vi "TW Convert Top Level.vi"() -> ()   [LabVIEW 2021, in "Plugin Generator.lvlib"]
uses:
  Plugin Generator.lvlib
panel:
  out "error out":errorcluster
  in  "Text color":u32(colorbox)
  in  "Background":u32(colorbox)=14457856
  in  "New Name":string="CIFRocks"
  in  "Template Project Path":path=path "D:/dev/Plugins/CIF_ROCKS/Tests/Template Interactive Test.lvproj"
  in  "Icon Text":string="RK-ON"
  # "To do:\nUpdate UI proj (will break after update)\nUpdate OOB test project\nUpdate Build Library project"
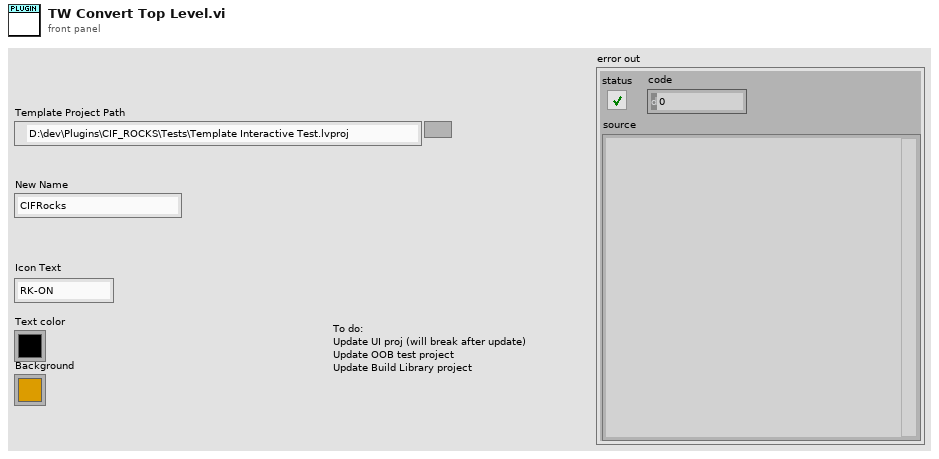
[diagram p1: front panel]
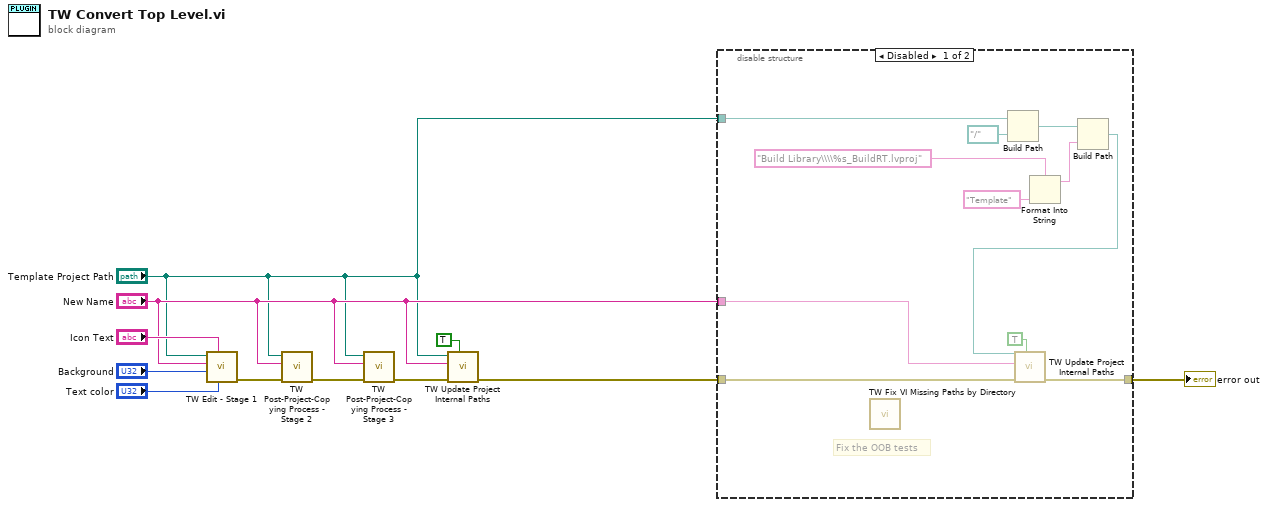
[diagram p0: block diagram]
diagram:
  n1 = call "TW Edit - Stage 1.vi"("Text color"="Text color", "Icon Text"="Icon Text", "Background"="Background", "New Subname"="New Name", "Template Project Path"="Template Project Path") -> ("error out"=w8:errorcluster)  [unwired: 5 in, 1 out]
  n2 = call "TW Post-Project-Copying Process - Stage 2.vi"("error in"=w8, "New Subname"="New Name", "Template Project Path"="Template Project Path") -> ("error out"=w7:errorcluster)  [unwired: 8 in]
  n3 = call "TW Post-Project-Copying Process - Stage 3.vi"("error in"=w7, "New Subname"="New Name", "Template Project Path"="Template Project Path") -> ("error out"=w6:errorcluster)  [unwired: 8 in]
  n4 = call "TW Update Project Internal Paths.vi"("Rename Project"=TRUE, "error in (no error)"=w6, "New Subname"="New Name", "Project Path"="Template Project Path") -> ("error out"=w4:errorcluster)  [unwired: 7 in]
  n5 = disable-structure shown="Disabled" {
    disable-tunnel: w4 -> [w22 w23]
    disable-tunnel: "New Name" -> [w21 _]
    disable-tunnel: [w12 w23] -> w2
    disable-tunnel: "Template Project Path" -> [w14 _]
    frame Disabled {
      # "Fix the OOB tests"
      n6 = call "TW Fix VI Missing Paths by Directory.vi"() -> ()  [unwired: 11 in, 1 out]
      n7 = Build Path(base path=w14, name or relative path=path "../..") -> (appended path=w16:path)
      n8 = Format Into String(format string="Build Library\\\\%s_BuildRT.lvproj" ("Class Name"), "Template" ("input 1")) -> (resulting string=w19:string)  [unwired: 2 in, 1 out]
      n9 = Build Path(base path=w16, name or relative path=w19) -> (appended path=w13:path)
      n10 = call "TW Update Project Internal Paths.vi"("Rename Project"=TRUE, "error in (no error)"=w22, "New Subname"=w21, "Project Path"=w13) -> ("error out"=w12:errorcluster)  [unwired: 7 in]
    }
    frame Enabled {
    }
  }
  "error out" <- w2
